vi "MotorController.vi"() -> ()   [LabVIEW 2012]
uses:
  <vilib>/robotics/Steering/Mecanum Steering Frame/NI_Robotics_Mecanum Steering Frame.lvclass
  <vilib>/robotics/Steering/Steering Frame/Apply Steering Frame Velocity to Wheels.vi
  <vilib>/Utility/error.llb/Error Cluster From Error Code.vi
  <vilib>/rvi/errors/niLvFpgaAdjustHostInterfaceError.vi
  <vilib>/rvi/interface/nirviReadWriteControl/nirviReadWriteControl.xnode
  <vilib>/robotics/Steering/Steering Frame/NI_Robotics_Steering Frame.lvclass
  NiFpgaLv.dll
  <vilib>/rvi/interface/Simulation/niFpgaSimulationCallBeginRW.vi
panel:
  out "error out 2":errorcluster
  out "steering frame out":refnum<class "NI_Robotics_Mecanum Steering Frame.lvclass">
  in  "error out":errorcluster
  in  "mecanum steering frame out":refnum<class "NI_Robotics_Mecanum Steering Frame.lvclass">
  in  "FPGA VI Reference In":refnum<k20>
  in  "Enable":bool
  out "Front Left":dbl format="%#.2g"
  out "Front Right":dbl format="%#.2g"
  out "Rear Left":dbl format="%#.2g"
  out "Rear Right":dbl format="%#.2g"
  in  "X Velocity (m/s)":dbl(slide) min=-1.0 max=1.0 scale=-1.0..1.0
  in  "Y Velocity (m/s)":dbl(slide) min=-1.0 max=1.0 scale=-1.0..1.0
  in  "Angular Velocity (rad/s)":dbl(slide) min=-1.0 max=1.0 scale=1.0..-1.0
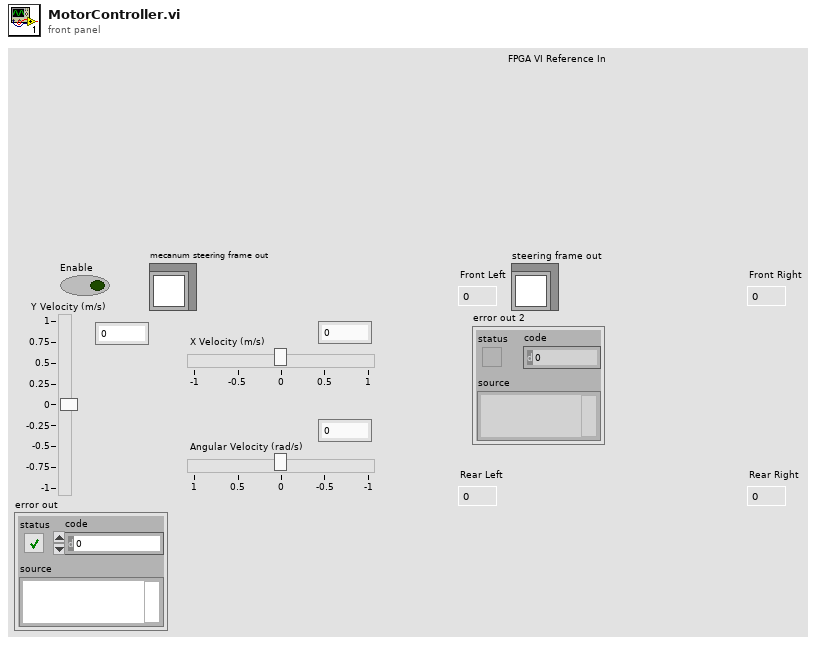
[diagram p1: front panel]
types:
  T1 = typedef "NI_Robotics_Wheel.lvclass/Wheel State.ctl" = cluster{"wheel name":string, "forward angular velocity":dbl, "caster angular velocity":dbl, "caster wheel angle (rad)":dbl, "steering angle (rad)":dbl}
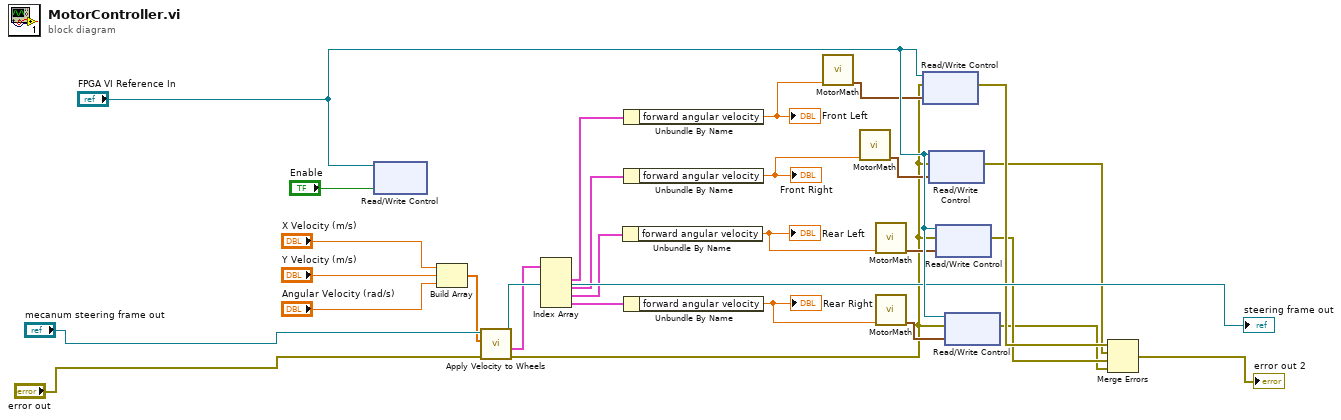
[diagram p0: block diagram]
diagram:
  n1 = xnode "Read/Write Control"("FPGA VI Reference In"="FPGA VI Reference In", "Enable"="Enable") -> ()  [unwired: 1 in, 2 out]
  n2 = Build Array("X Velocity (m/s)", "Y Velocity (m/s)", "Angular Velocity (rad/s)") -> (w20:dbl[])
  n3 = call-poly <vilib>:"Apply Velocity to Wheels.vi"("error in (no error)"="error out", "steering frame velocity"=w20, "steering frame in"="mecanum steering frame out") -> ("error out"=w6:errorcluster, "calculated wheel states"=w19:T1[], "steering frame out"=→"steering frame out":refnum<class "NI_Robotics_Mecanum Steering Frame.lvclass">)  [unwired: 5 in, 1 out]
  n4 = Index Array(array=w19) -> (element #1=w18:T1, element #2=w17:T1, element #3=w16:T1, element #4=w22:T1)  [unwired: 4 in]
  n5 = Unbundle By Name(w16) -> ("forward angular velocity"=w9:dbl)
  "Rear Left" <- w9
  n6 = Unbundle By Name(w18) -> ("forward angular velocity"=w15:dbl)
  "Front Left" <- w15
  n7 = Unbundle By Name(w17) -> ("forward angular velocity"=w10:dbl)
  "Front Right" <- w10
  n8 = Unbundle By Name(w22) -> ("forward angular velocity"=w8:dbl)
  "Rear Right" <- w8
  n9 = call "MotorMath.vi"("x"=w15) -> ("output cluster"=w14:cluster{i32, "upper limit":dbl})  [unwired: 10 in]
  n10 = call "MotorMath.vi"("x"=w10) -> ("output cluster"=w13:cluster{i32, "upper limit":dbl})  [unwired: 10 in]
  n11 = call "MotorMath.vi"("x"=w9) -> ("output cluster"=w12:cluster{i32, "upper limit":dbl})  [unwired: 10 in]
  n12 = call "MotorMath.vi"("x"=w8) -> ("output cluster"=w11:cluster{i32, "upper limit":dbl})  [unwired: 10 in]
  n13 = xnode "Read/Write Control"("FPGA VI Reference In"="FPGA VI Reference In", "error in"=w6, "Motor 1"=w14) -> ("error out"=w5:errorcluster)  [unwired: 1 out]
  n14 = xnode "Read/Write Control"("FPGA VI Reference In"="FPGA VI Reference In", "error in"=w6, "Motor 2"=w13) -> ("error out"=w4:errorcluster)  [unwired: 1 out]
  n15 = xnode "Read/Write Control"("FPGA VI Reference In"="FPGA VI Reference In", "error in"=w6, "Motor 3"=w12) -> ("error out"=w3:errorcluster)  [unwired: 1 out]
  n16 = xnode "Read/Write Control"("FPGA VI Reference In"="FPGA VI Reference In", "error in"=w6, "Motor 4"=w11) -> ("error out"=w2:errorcluster)  [unwired: 1 out]
  n17 = Merge Errors(w5, w4, w3, w2) -> (→"error out 2":errorcluster)
